vi "ClimberExtend.vi"   [LabVIEW 2020]
uses:
  Swerve Global Variables.vi
  Robot Global Data.vi
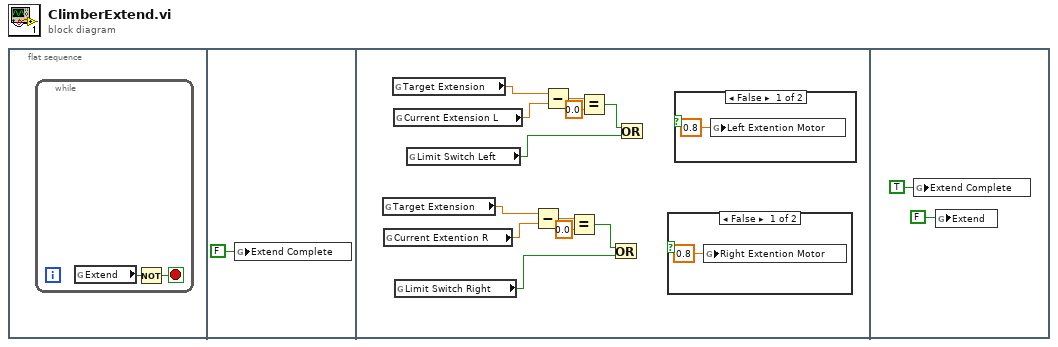
[diagram p0: block diagram]
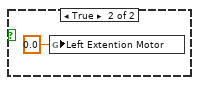
[diagram p2: hidden frame]
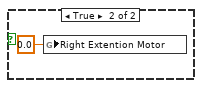
[diagram p3: hidden frame]
diagram:
  n1 = flat-sequence {
    frame #0 {
      n2 = while {
        stop <- w2 stop-if-true
        n3 = global read "Robot Global Data.vi" "Extend"() -> (w1:bool)
        n4 = Not(x=w1) -> (.not. x?=w2:bool)
      }
    }
    frame #1 {
      n5 = global write "Robot Global Data.vi" "Extend Complete"(FALSE ("Extend Complete")) -> ()
    }
    frame #2 {
      n6 = global read "Swerve Global Variables.vi" "Target Extension"() -> (w11:dbl)
      n7 = global read "Swerve Global Variables.vi" "Current Extention R"() -> (w10:dbl)
      n8 = global read "Swerve Global Variables.vi" "Target Extension"() -> (w15:dbl)
      n9 = global read "Swerve Global Variables.vi" "Current Extension L"() -> (w14:dbl)
      n10 = global read "Robot Global Data.vi" "Limit Switch Right"() -> (w4:bool)
      n11 = global read "Robot Global Data.vi" "Limit Switch Left"() -> (w6:bool)
      n12 = Subtract(x=w11, y=w10) -> (x-y=w9:dbl)
      n13 = Subtract(x=w15, y=w14) -> (x-y=w13:dbl)
      n14 = Equal?(x=w9, y=0.0) -> (x = y?=w5:bool)
      n15 = Equal?(x=w13, y=0.0) -> (x = y?=w7:bool)
      n16 = Or(x=w5, y=w4) -> ()  [unwired: 1 out]
      n17 = Or(x=w7, y=w6) -> ()  [unwired: 1 out]
      n18 = case shown="False" {
        selector: _ -> [_ _]
        frame False {
          n19 = global write "Swerve Global Variables.vi" "Right Extention Motor"(0.8 ("Right Extention Motor")) -> ()
        }
        frame True {
          n20 = global write "Swerve Global Variables.vi" "Right Extention Motor"(0.0 ("Right Extention Motor")) -> ()
        }
      }
      n21 = case shown="False" {
        selector: _ -> [_ _]
        frame False {
          n22 = global write "Swerve Global Variables.vi" "Left Extention Motor"(0.8 ("Left Extention Motor")) -> ()
        }
        frame True {
          n23 = global write "Swerve Global Variables.vi" "Left Extention Motor"(0.0 ("Left Extention Motor")) -> ()
        }
      }
    }
    frame #3 {
      n24 = global write "Robot Global Data.vi" "Extend Complete"(TRUE ("Extend Complete")) -> ()
      n25 = global write "Robot Global Data.vi" "Extend"(FALSE ("Extend Complete")) -> ()
    }
  }
